vi "Car Wash Server.vi"() -> ()   [LabVIEW 2024]
uses:
  <vilib>/Utility/file.llb/Read Delimited Spreadsheet (string).vi
panel:
  in  "Data Loging":string[][](table)
  in  "User Data":string[][](table)
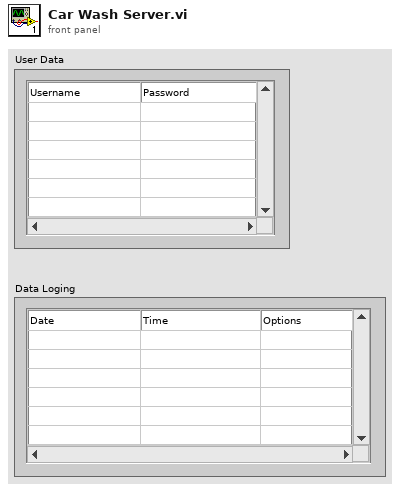
[diagram p1: front panel]
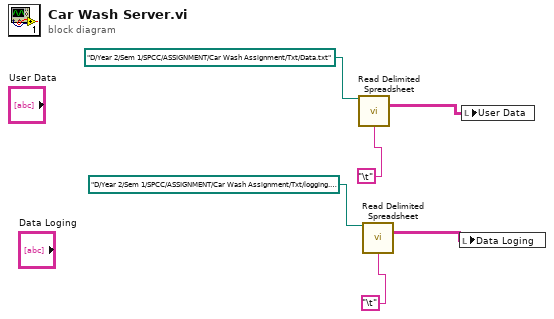
[diagram p0: block diagram]
diagram:
  n1 = call-poly <vilib>:"Read Delimited Spreadsheet.vi"("file path (dialog if empty)"=path "D:/Year 2/Sem 1/SPCC/ASSIGNMENT/Car Wash Assignment/Txt/Data.txt", "delimiter (\\t)"="\t") -> ("all rows"=w5:string[][])  [unwired: 8 in, 5 out]
  n2 = call-poly <vilib>:"Read Delimited Spreadsheet.vi"("file path (dialog if empty)"=path "D:/Year 2/Sem 1/SPCC/ASSIGNMENT/Car Wash Assignment/Txt/logging.txt", "delimiter (\\t)"="\t") -> ("all rows"=w2:string[][])  [unwired: 8 in, 5 out]
  n3 = local write "Data Loging"(w2) -> ()
  n4 = local write "User Data"(w5) -> ()
